vi "ConfirmReceipt.vi"(8 "error in (no error)":errorcluster, 9 "timeout in ms (10000)":i32=10000, 11 "STOMP in":refnum<class "STOMP.lvclass">) -> (0 "error out":errorcluster, 3 "STOMP out":refnum<class "STOMP.lvclass">)   [LabVIEW 2017, in "STOMP.lvclass"]
uses:
  STOMP.lvclass
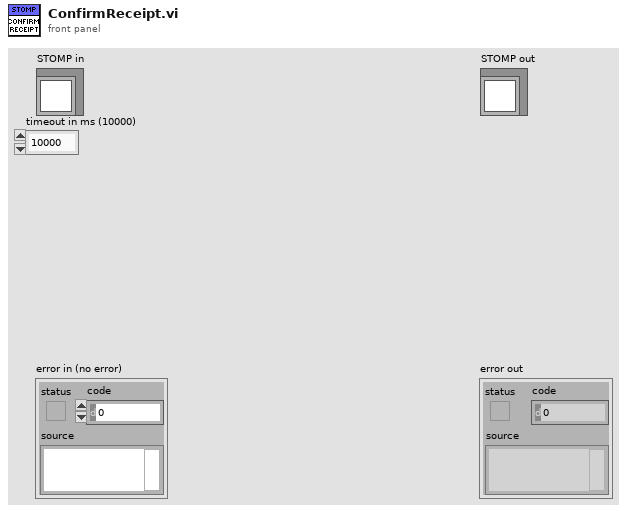
[diagram p1: front panel]
types:
  T1 = typedef "STOMP.lvclass/ObjectAttributes.ctl" = cluster{"address":string, "port":u16, "ConnectionRef":refnum<k5>, "messageQueue":refnum<queue>, "receiptQueue":refnum<queue>, "errorQueue":refnum<queue>, "sendQueue":refnum<queue>, "currentReceiptNumber":u64, "currentSubscriptionId":u64, "closeConnection":bool, "activeSubscriptions":T2[]}
  T2 = typedef "STOMP.lvclass/Type_ActiveSubscription.ctl" = cluster{"id":u64, "receipt":bool, "Destination":string, "ack":T3, "headers":T4[]}
  T3 = typedef "STOMP.lvclass/Type_AckHeader.ctl" = enum16{"auto", "client", "client-individual"}
  T4 = typedef "STOMP.lvclass/Type_FrameHeader.ctl" = cluster{"Header":string, "Value":string}
  T5 = typedef "STOMP.lvclass/Type_ServerFrame.ctl" = cluster{"Type":T6, "Headers":cluster{"Header":string, "Value":string}[], "Body":string}
  T6 = typedef "STOMP.lvclass/Type_ServerFrameType.ctl" = enum16{"Undefined", "MESSAGE", "CONNECTED", "RECEIPT", "ERROR"}
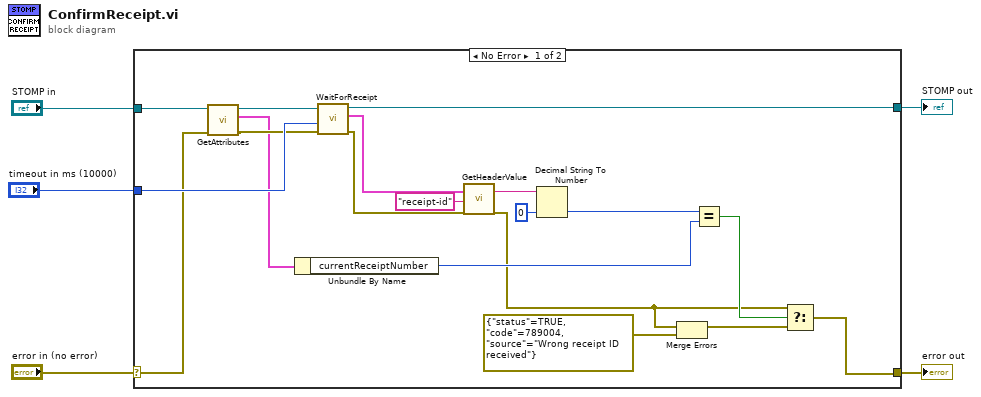
[diagram p0: block diagram]
diagram:
  n1 = case shown="No Error" "error in (no error)" {
    selector: "error in (no error)" -> [w10 w26]
    tunnel: [w11 w26] -> w4
    tunnel: [w19 w25] -> w2
    tunnel: "STOMP in" -> [w9 w25]
    tunnel: "timeout in ms (10000)" -> [w16 _]
    frame No Error {
      n2 = call-dynamic "GetAttributes.vi"("error in (no error)"=w10, "STOMP in"=w9) -> ("error out"=w7:errorcluster, "attributes"=w6:T1, "STOMP out"=w8:refnum<class "STOMP.lvclass">)  [unwired: 7 in]
      n3 = Unbundle By Name(w6) -> ("currentReceiptNumber"=w18:u64)
      n4 = call-dynamic "WaitForReceipt.vi"("error in (no error)"=w7, "timeout in ms (10000)"=w16, "STOMP in"=w8) -> ("error out"=w23:errorcluster, "receipt"=w24:T5, "STOMP out"=w19:refnum<class "STOMP.lvclass">)  [unwired: 6 in]
      n5 = call "GetHeaderValue.vi"("Server Frame"=w24, "Header Name"="receipt-id", "error in"=w23) -> ("Value"=w21:string, "error out"=w14:errorcluster)  [unwired: 14 in, 1 out]
      n6 = Decimal String To Number(string=w21, default (0L)=u64 0 ("default (0 I32)")) -> (number=w17:u64)  [unwired: 1 in, 1 out]
      n7 = Merge Errors(w14, errorcluster {"status"=TRUE, "code"=789004, "source"="Wrong receipt ID received"} ("error in")) -> (w12:errorcluster)
      n8 = Equal?(x=w17, y=w18) -> (x = y?=w15:bool)
      n9 = Select(t=w14, s=w15, f=w12) -> (s? t:f=w11:errorcluster)
    }
    frame Error {
    }
  }
  "error out" <- w4
  "STOMP out" <- w2
